vi "Parse-attribute.vi"(8 "error in (no error)":errorcluster, 10 "String in":string, 11 "Coordinate in":refnum<class "Coordinate.lvclass">) -> (0 "error out":errorcluster, 1 "Valid attribute?":bool, 2 "Remaining string":string, 3 "Coordinate out":refnum<class "Coordinate.lvclass">)   [LabVIEW 2013, in "MaterialCharacterization.lvlib" / "Coordinate.lvclass"]
uses:
  Coordinate.lvclass
  Coordinate.lvclass/Coordinate.ctl
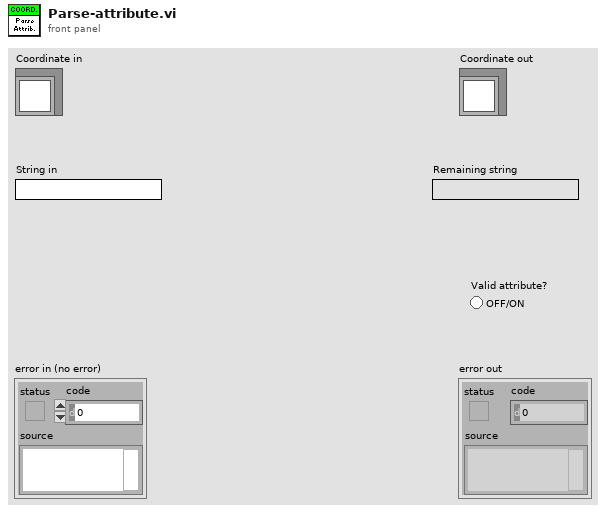
[diagram p1: front panel]
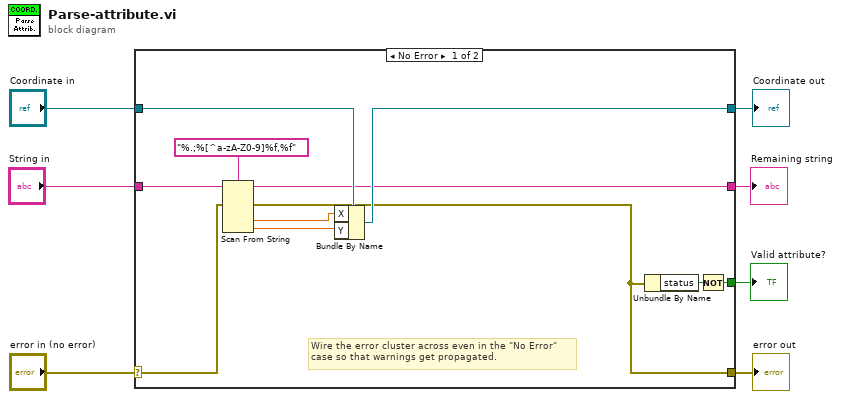
[diagram p0: block diagram]
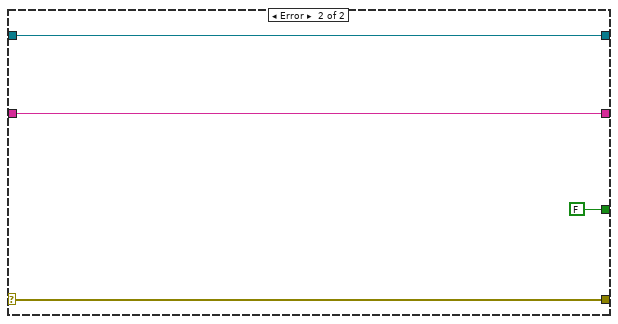
[diagram p2: hidden frame]
diagram:
  n1 = case shown="No Error" "error in (no error)" {
    selector: "error in (no error)" -> [w13 w22]
    tunnel: [w8 w22] -> w6
    tunnel: [w11 w21] -> w4
    tunnel: "Coordinate in" -> [w12 w21]
    tunnel: "String in" -> [w14 w19]
    tunnel: [w10 w19] -> w2
    tunnel: [w9 FALSE] -> w1
    frame No Error {
      # "Wire the error cluster across even in the \"No Error\"\ncase so that warnings get propagated."
      n2 = Scan From String(format string="%.;%[^a-zA-Z0-9]%f,%f", input string=w14, error in=w13) -> (remaining string=w10:string, error out=w8:errorcluster, output 2=w16:dbl, output 3=w15:dbl)  [unwired: 5 in, 1 out]
      n3 = Bundle By Name(cluster=w12, "X"=w16, "Y"=w15) -> (w11:refnum<class "Coordinate.lvclass">)
      n4 = Unbundle By Name(w8) -> ("status"=w17:bool)
      n5 = Not(x=w17) -> (.not. x?=w9:bool)
    }
    frame Error {
    }
  }
  "error out" <- w6
  "Coordinate out" <- w4
  "Remaining string" <- w2
  "Valid attribute?" <- w1
